vi "getViConPane.vi"(8 "error in (no error)":errorcluster, 11 "VI in":refnum<vi>) -> (0 "error out":errorcluster, 2 "Connector Pane Patterns":T1=3, 3 "VI out":refnum<vi>)   [LabVIEW 2017, in "vi_tools.lvlib"]
uses:
  vi_tools.lvlib
  connectorPanePatterns.ctl
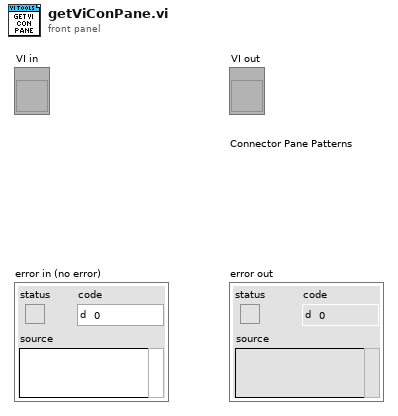
[diagram p1: front panel]
types:
  T1 = typedef "vi_tools.lvlib/connectorPanePatterns.ctl" = i32
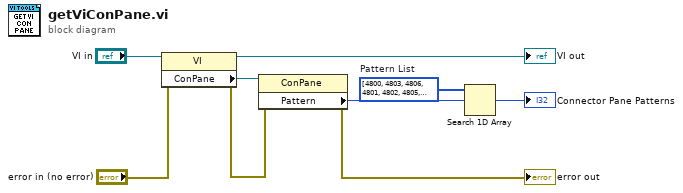
[diagram p0: block diagram]
diagram:
  w3 = u32[] [4800, 4803, 4806, 4801, 4802, 4805, 4830, 4804, 4807, 4831, 4832, 4810, 4808, 4809, 4811, 4812, 4816, 4823, 4824, 4817, 4818, 4825, 4819, 4813, 4820, 4826, 4821, 4827, 4828, 4822, 4814, 4829, 4815, 4833, 4834, 4835]  # Pattern List
  n1 = property class="VI"(reference="VI in", error in="error in (no error)") -> (reference out=→"VI out":refnum<vi>, error out=w8:errorcluster, "ConPane"=w7:refnum<vi>)
  n2 = property class="ConPane"(reference=w7, error in=w8) -> (error out=→"error out":errorcluster, "Pattern"=w2:u32)  [unwired: 1 out]
  n3 = Search 1D Array(1D array=w3, element=w2) -> (index of element=→"Connector Pane Patterns":i32)  [unwired: 1 in]
